vi "VirtualJoyStick.vi"(0 "In Contact":refnum<vi>, 1 "Status":refnum<vi>, 2 "Jog (um) raise":dbl, 3 "Jog (um)":dbl, 4 "Position 1":i32[](array[numeric]), 5 "Motor Zero":refnum<vi>, 6 "Steps Per micron":dbl, 7 "JoyStickRefs 2":T1) -> ()   [LabVIEW 2020]
uses:
  C:/Projects/RaxTagServer/LabviewDXFViewer/LabviewDXFViewer/bin/Release/LabviewDXFViewer.exe
  LabviewDXFViewer/bin/Release/LabviewDXFViewer.exe
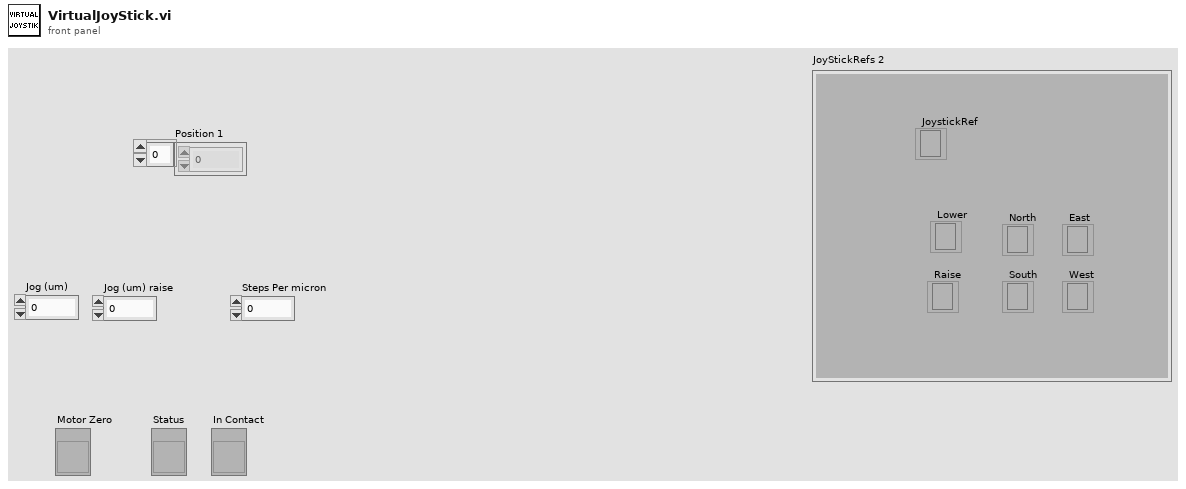
[diagram p1: front panel]
types:
  T1 = cluster{"North":refnum<k24>, "South":refnum<k24>, "Lower":refnum<k24>, "Raise":refnum<k24>, "JoystickRef":refnum<k24>, "West":refnum<k24>, "East":refnum<k24>}
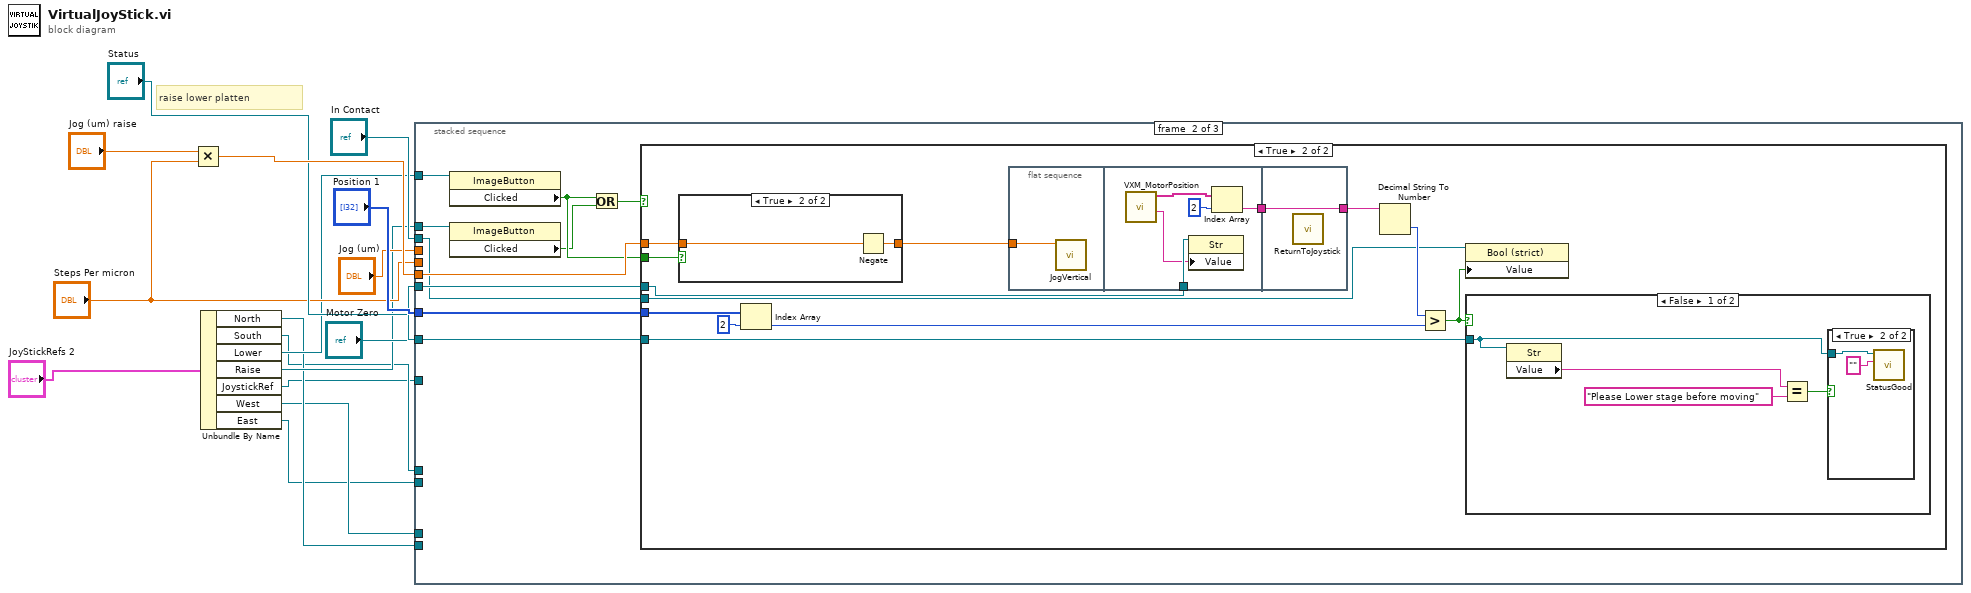
[diagram p0: block diagram]
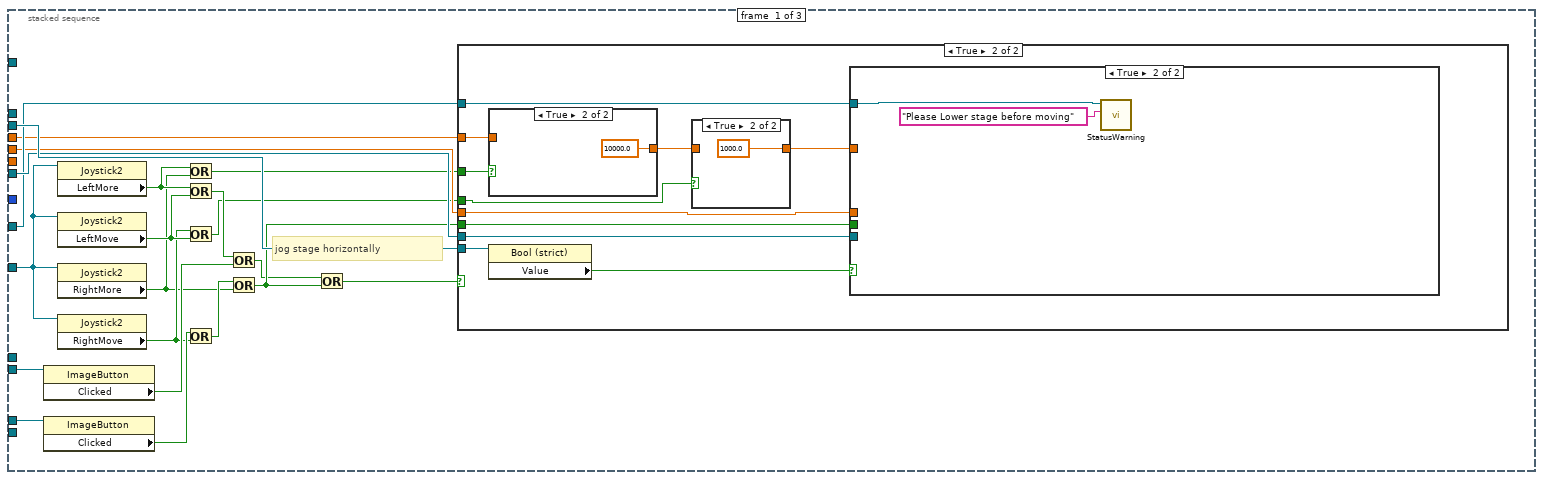
[diagram p2: hidden frame]
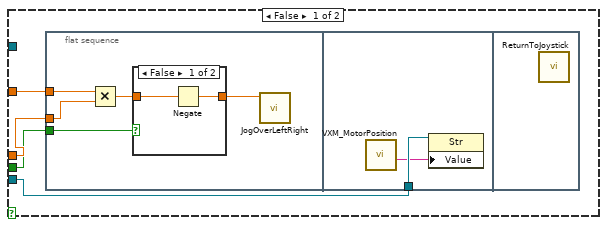
[diagram p4: hidden frame]
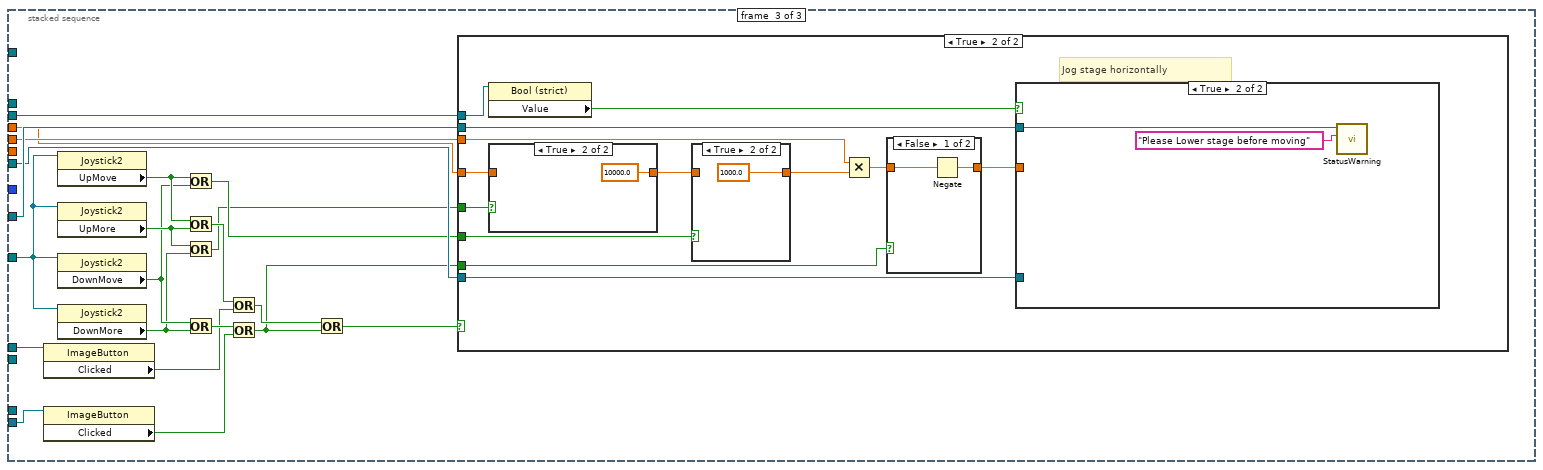
[diagram p12: hidden frame]
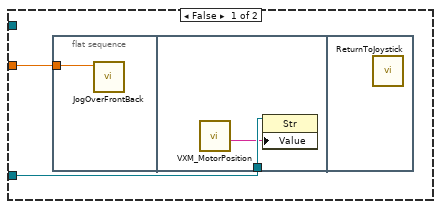
[diagram p14: hidden frame]
diagram:
  # "raise lower platten"
  n1 = Multiply(x="Jog (um) raise", y="Steps Per micron") -> (x*y=w15:dbl)
  n2 = Unbundle By Name("JoyStickRefs 2") -> ("North"=w6:refnum<k24>, "South"=w5:refnum<k24>, "Lower"=w8:refnum<k24>, "Raise"=w7:refnum<k24>, "JoystickRef"=w2:refnum<k24>, "West"=w4:refnum<k24>, "East"=w3:refnum<k24>)
  n3 = stacked-sequence {
    tunnel: w15 -> [_ w78 _]
    tunnel: "Position 1" -> [_ w76 _]
    tunnel: "Status" -> [w35 w69 w128]
    tunnel: "In Contact" -> [w37 w75 w127]
    tunnel: "Steps Per micron" -> [w33 _ w126]
    tunnel: "Jog (um)" -> [w34 _ w125]
    tunnel: "Motor Zero" -> [w36 w77 w124]
    tunnel: w8 -> [_ w73 _]
    tunnel: w7 -> [_ w71 _]
    tunnel: w6 -> [_ _ w116]
    tunnel: w5 -> [_ _ w114]
    tunnel: w4 -> [w24 _ _]
    tunnel: w3 -> [w22 _ _]
    tunnel: w2 -> [w20 _ w112]
    frame #0 {
      # "jog stage horizontally"
      n4 = property class="ImageButton"(reference=w22) -> ("Clicked"=w21:bool)  [unwired: 1 in, 2 out]
      n5 = property class="ImageButton"(reference=w24) -> ("Clicked"=w23:bool)  [unwired: 1 in, 2 out]
      n6 = property class="Joystick2"(reference=w20) -> ("LeftMore"=w18:bool)  [unwired: 1 in, 2 out]
      n7 = property class="Joystick2"(reference=w20) -> ("LeftMove"=w25:bool)  [unwired: 1 in, 2 out]
      n8 = property class="Joystick2"(reference=w20) -> ("RightMore"=w17:bool)  [unwired: 1 in, 2 out]
      n9 = property class="Joystick2"(reference=w20) -> ("RightMove"=w19:bool)  [unwired: 1 in, 2 out]
      n10 = Or(x=w18, y=w17) -> (x .or. y?=w27:bool)
      n11 = Or(x=w18, y=w25) -> (x .or. y?=w28:bool)
      n12 = Or(x=w19, y=w25) -> (x .or. y?=w26:bool)
      n13 = Or(x=w23, y=w19) -> (x .or. y?=w30:bool)
      n14 = Or(x=w28, y=w21) -> (x .or. y?=w29:bool)
      n15 = Or(x=w30, y=w17) -> (x .or. y?=w31:bool)
      n16 = Or(x=w29, y=w31) -> (x .or. y?=w32:bool)
      n17 = case shown="True" w32 {
        tunnel: w34 -> [_ w45]
        tunnel: w33 -> [_ w48]
        tunnel: w27 -> [_ w47]
        tunnel: w31 -> [_ w43]
        tunnel: w26 -> [_ w42]
        tunnel: w36 -> [_ w41]
        tunnel: w35 -> [_ w40]
        tunnel: w37 -> [_ w39]
        frame False {
        }
        frame True {
          n18 = case shown="True" w47 {
            tunnel: [w67 10000.0 ("Jog (um)")] -> w44
            tunnel: w45 -> [w67 _]
            frame False {
            }
            frame True {
            }
          }
          n19 = property class="Bool (strict)"(reference=w39) -> ("Value"=w38:bool)  [unwired: 1 in, 2 out]
          n20 = case shown="True" w42 {
            tunnel: [w65 1000.0 ("Jog (um)")] -> w46
            tunnel: w44 -> [w65 _]
            frame False {
            }
            frame True {
            }
          }
          n21 = case shown="True" w38 {
            tunnel: w48 -> [w52 _]
            tunnel: w46 -> [w51 _]
            tunnel: w43 -> [w50 _]
            tunnel: w41 -> [w49 _]
            tunnel: w40 -> [_ w63]
            frame False {
              n22 = flat-sequence {
                tunnel: w52 -> [w55]
                tunnel: w51 -> [w54]
                tunnel: w50 -> [w53]
                tunnel: w49 -> [w62]
                frame #0 {
                  n23 = Multiply(x=w54, y=w55) -> (x*y=w56:dbl)
                  n24 = case shown="False" w53 {
                    tunnel: [w58 w60] -> w57
                    tunnel: w56 -> [w59 w60]
                    frame False {
                      n25 = Negate(x=w59) -> (-x=w58:dbl)
                    }
                    frame True {
                    }
                  }
                  n26 = call "JogOverLeftRight.vi"("Numeric"=w57) -> ()  [unwired: 11 in]
                }
                frame #1 {
                  n27 = call "VXM_MotorPosition.vi"() -> ("Position String"=w61:string)  [unwired: 10 in, 1 out]
                  n28 = property class="Str"(reference=w62, "Value"=w61) -> ()  [unwired: 1 in, 2 out]
                }
                frame #2 {
                  n29 = call "ReturnToJoystick.vi"() -> ()  [unwired: 12 in]
                }
              }
            }
            frame True {
              n30 = call "StatusWarning.vi"("Text.Text"="Please Lower stage before moving" ("Status"), "String in"=w63) -> ()  [unwired: 10 in]
            }
          }
        }
      }
    }
    frame #1 {
      n31 = property class="ImageButton"(reference=w73) -> ("Clicked"=w72:bool)  [unwired: 1 in, 2 out]
      n32 = property class="ImageButton"(reference=w71) -> ("Clicked"=w70:bool)  [unwired: 1 in, 2 out]
      n33 = Or(x=w72, y=w70) -> (x .or. y?=w74:bool)
      n34 = case shown="True" w74 {
        tunnel: w72 -> [_ w91]
        tunnel: w78 -> [_ w89]
        tunnel: w77 -> [_ w84]
        tunnel: w76 -> [_ w83]
        tunnel: w75 -> [_ w82]
        tunnel: w69 -> [_ w79]
        frame False {
        }
        frame True {
          n35 = case shown="True" w91 {
            tunnel: [w105 w106] -> w90
            tunnel: w89 -> [w105 w107]
            frame False {
            }
            frame True {
              n36 = Negate(x=w107) -> (-x=w106:dbl)
            }
          }
          n37 = Index Array(array=w83, index=2) -> (element=w86:i32)
          n38 = flat-sequence {
            tunnel: w90 -> [w98]
            tunnel: w84 -> [w103]
            tunnel: [w99] -> w81
            tunnel: [w104] -> w88
            tunnel: w81 -> [w104]
            frame #0 {
              n39 = call "JogVertical.vi"("Numeric"=w98) -> ()  [unwired: 11 in]
            }
            frame #1 {
              n40 = call "VXM_MotorPosition.vi"() -> ("Position String"=w102:string, "Array"=w101:string[])  [unwired: 10 in]
              n41 = property class="Str"(reference=w103, "Value"=w102) -> ()  [unwired: 1 in, 2 out]
              n42 = Index Array(array=w101, index=2) -> (element=w99:string)
            }
            frame #2 {
              n43 = call "ReturnToJoystick.vi"() -> ()  [unwired: 12 in]
            }
          }
          n44 = Decimal String To Number(string=w88) -> (number=w87:i32)  [unwired: 2 in, 1 out]
          n45 = Greater?(x=w87, y=w86) -> (0:w80:bool)
          n46 = property class="Bool (strict)"(reference=w82, "Value"=w80) -> ()  [unwired: 1 in, 2 out]
          n47 = case shown="False" w80 {
            tunnel: w79 -> [w92 _]
            frame False {
              n48 = property class="Str"(reference=w92) -> ("Value"=w95:string)  [unwired: 1 in, 2 out]
              n49 = Equal?(x=w95, y="Please Lower stage before moving" ("Status")) -> (x = y?=w93:bool)
              n50 = case shown="True" w93 {
                tunnel: w92 -> [_ w97]
                frame False {
                }
                frame True {
                  n51 = call "StatusGood.vi"("Text.Text"="", "String in"=w97) -> ()  [unwired: 10 in]
                }
              }
            }
            frame True {
            }
          }
        }
      }
    }
    frame #2 {
      n52 = property class="ImageButton"(reference=w114) -> ("Clicked"=w113:bool)  [unwired: 1 in, 2 out]
      n53 = property class="ImageButton"(reference=w116) -> ("Clicked"=w115:bool)  [unwired: 1 in, 2 out]
      n54 = property class="Joystick2"(reference=w112) -> ("UpMove"=w111:bool)  [unwired: 1 in, 2 out]
      n55 = property class="Joystick2"(reference=w112) -> ("UpMore"=w110:bool)  [unwired: 1 in, 2 out]
      n56 = property class="Joystick2"(reference=w112) -> ("DownMove"=w109:bool)  [unwired: 1 in, 2 out]
      n57 = property class="Joystick2"(reference=w112) -> ("DownMore"=w108:bool)  [unwired: 1 in, 2 out]
      n58 = Or(x=w111, y=w109) -> (x .or. y?=w118:bool)
      n59 = Or(x=w111, y=w110) -> (x .or. y?=w120:bool)
      n60 = Or(x=w110, y=w108) -> (x .or. y?=w117:bool)
      n61 = Or(x=w109, y=w108) -> (x .or. y?=w119:bool)
      n62 = Or(x=w120, y=w113) -> (x .or. y?=w122:bool)
      n63 = Or(x=w119, y=w115) -> (x .or. y?=w121:bool)
      n64 = Or(x=w122, y=w121) -> (x .or. y?=w123:bool)
      n65 = case shown="True" w123 {
        tunnel: w121 -> [_ w141]
        tunnel: w117 -> [_ w139]
        tunnel: w118 -> [_ w137]
        tunnel: w128 -> [_ w134]
        tunnel: w127 -> [_ w133]
        tunnel: w126 -> [_ w131]
        tunnel: w125 -> [_ w130]
        tunnel: w124 -> [_ w129]
        frame False {
        }
        frame True {
          # "Jog stage horizontally"
          n66 = property class="Bool (strict)"(reference=w133) -> ("Value"=w132:bool)  [unwired: 1 in, 2 out]
          n67 = case shown="True" w139 {
            tunnel: [w151 10000.0 ("Jog (um)")] -> w136
            tunnel: w130 -> [w151 _]
            frame False {
            }
            frame True {
            }
          }
          n68 = case shown="True" w137 {
            tunnel: [w149 1000.0 ("Jog (um)")] -> w135
            tunnel: w136 -> [w149 _]
            frame False {
            }
            frame True {
            }
          }
          n69 = Multiply(x=w131, y=w135) -> (x*y=w138:dbl)
          n70 = case shown="False" w141 {
            tunnel: [w153 w155] -> w140
            tunnel: w138 -> [w154 w155]
            frame False {
              n71 = Negate(x=w154) -> (-x=w153:dbl)
            }
            frame True {
            }
          }
          n72 = case shown="True" w132 {
            tunnel: w140 -> [w143 _]
            tunnel: w134 -> [_ w147]
            tunnel: w129 -> [w142 _]
            frame False {
              n73 = flat-sequence {
                tunnel: w143 -> [w144]
                tunnel: w142 -> [w146]
                frame #0 {
                  n74 = call "JogOverFrontBack.vi"("Numeric"=w144) -> ()  [unwired: 11 in]
                }
                frame #1 {
                  n75 = call "VXM_MotorPosition.vi"() -> ("Position String"=w145:string)  [unwired: 10 in, 1 out]
                  n76 = property class="Str"(reference=w146, "Value"=w145) -> ()  [unwired: 1 in, 2 out]
                }
                frame #2 {
                  n77 = call "ReturnToJoystick.vi"() -> ()  [unwired: 12 in]
                }
              }
            }
            frame True {
              n78 = call "StatusWarning.vi"("Text.Text"="Please Lower stage before moving" ("Status"), "String in"=w147) -> ()  [unwired: 10 in]
            }
          }
        }
      }
    }
  }
